vi "Volt to C.vi"(11 "Voltage":dbl) -> (2 "R (ohm)":dbl, 3 "interpolation value":dbl format="%0.2f")   [LabVIEW 2020]
uses:
  <vilib>/Analysis/NI_AALPro.lvlib
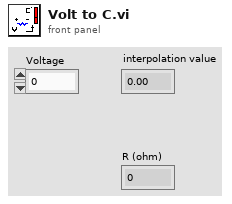
[diagram p1: front panel]
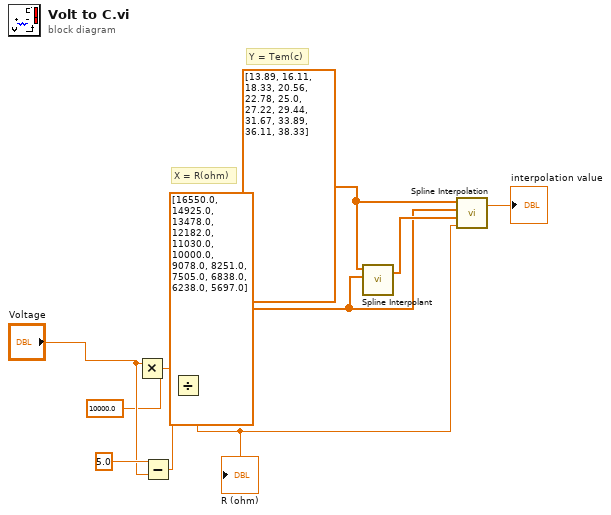
[diagram p0: block diagram]
diagram:
  w2 = dbl[] [13.89, 16.11, 18.33, 20.56, 22.78, 25.0, 27.22, 29.44, 31.67, 33.89, 36.11, 38.33]
  w1 = dbl[] [16550.0, 14925.0, 13478.0, 12182.0, 11030.0, 10000.0, 9078.0, 8251.0, 7505.0, 6838.0, 6238.0, 5697.0]
  # "Y = Tem(c)"
  # "X = R(ohm)"
  n1 = Multiply(x="Voltage", y=10000.0) -> (x*y=w6:dbl)
  n2 = Subtract(x=5.0, y="Voltage") -> (x-y=w9:dbl)
  n3 = Divide(x=w6, y=w9) -> (x/y=w10:dbl)
  "R (ohm)" <- w10
  n4 = call <vilib>:"Spline Interpolant.vi"("X"=w1, "Y"=w2) -> ("Interpolant"=w3:dbl[])  [unwired: 2 in, 1 out]
  n5 = call <vilib>:"Spline Interpolation.vi"("x value"=w10, "Interpolant"=w3, "X"=w1, "Y"=w2) -> ("interpolation value"=→"interpolation value":dbl)  [unwired: 1 out]
